vi "NumToTCANProperty.vi"(11 "TCANPropertyNum":u8) -> (3 "TCANProperty":T1)   [LabVIEW 2016]
uses:
  TCANProperty.ctl
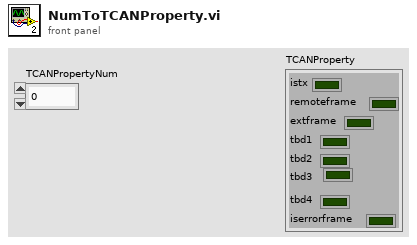
[diagram p1: front panel]
types:
  T1 = typedef "TCANProperty.ctl" = cluster{"istx":bool, "remoteframe":bool, "extframe":bool, "tbd1":bool, "tbd2":bool, "tbd3":bool, "tbd4":bool, "iserrorframe":bool}
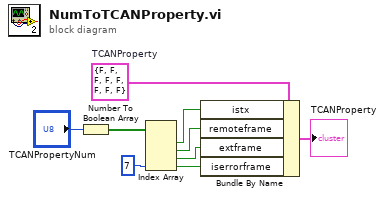
[diagram p0: block diagram]
diagram:
  w7 = T1 {"istx"=FALSE, "remoteframe"=FALSE, "extframe"=FALSE, "tbd1"=FALSE, "tbd2"=FALSE, "tbd3"=FALSE, "tbd4"=FALSE, "iserrorframe"=FALSE}  # TCANProperty
  n1 = Number To Boolean Array(number="TCANPropertyNum") -> (Boolean array=w9:bool[])
  n2 = Index Array(array=w9, index #4=7 ("索引")) -> (element #1=w3:bool, element #2=w4:bool, element #3=w5:bool, element #4=w6:bool)  [unwired: 3 in]
  n3 = Bundle By Name(cluster=w7, "istx"=w3, "remoteframe"=w4, "extframe"=w5, "iserrorframe"=w6) -> (→"TCANProperty":T1)
